vi "delete channel.vi"(10 "Sensor Array":T1, 11 "Indexvals in":u32) -> (2 "Sensor Array out":T1, 3 "Indexvals out":u32)   [LabVIEW 2010]
uses:
  DAQ configuration/Sensor array.ctl
  DAQ configuration/channel identifier.ctl
  global scale array.vi
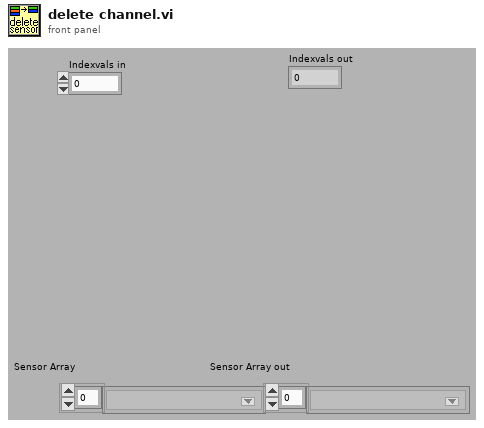
[diagram p1: front panel]
types:
  T1 = typedef "Sensor array.ctl" = T2[]
  T2 = typedef "channel identifier.ctl" = u16
  T3 = typedef "calib array.ctl" = T4[]
  T4 = typedef "conversion.ctl" = cluster{"conversion matrix":sgl[][], "units":string, "name":string, "scale type":T5, "offset (volts)":dbl, "second channel":i8, "correspondence table":T6, "offset (physical units)":dbl, "pH scale":T7, "D.O.":T8}
  T5 = typedef "scale type.ctl" = enum16{"Volts", "Polynomial", "Correspondence Table", "pH", "Dissolved Oxygen", "Quadratic"}
  T6 = typedef "correspondence table.ctl" = cluster{"physical units":dbl, "volts":dbl}[]
  T7 = typedef "pH scale.ctl" = cluster{"Buffers":cluster{"Buffer":dbl, "Calibrated":bool, "V/T":dbl}[], "Temperature":dbl}
  T8 = typedef "DO scale.ctl" = cluster{"Temperature":dbl, "K":dbl, "barometric pressure":dbl}
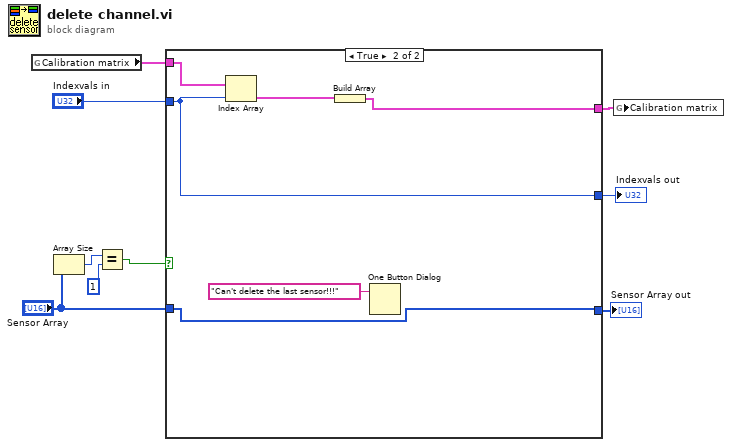
[diagram p0: block diagram]
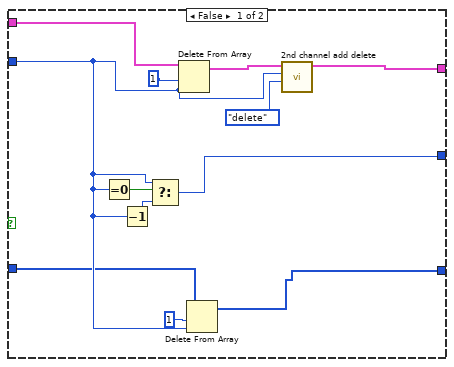
[diagram p2: hidden frame]
diagram:
  n1 = global read "global scale array.vi" "Calibration matrix"() -> (w2:T3)
  n2 = Array Size(array="Sensor Array") -> (size(s)=w6:i32)
  n3 = Equal?(x=w6, y=1) -> (x = y?=w4:bool)
  n4 = case shown="True" w4 {
    tunnel: "Indexvals in" -> [w16 w24]
    tunnel: [w14 w24] -> w8
    tunnel: "Sensor Array" -> [w13 w26]
    tunnel: [w12 w26] -> w3
    tunnel: w2 -> [w11 w25]
    tunnel: [w10 w22] -> w1
    frame False {
      n5 = Equal To 0?(x=w16) -> (x = 0?=w17:bool)
      n6 = Decrement(x=w16) -> (x-1=w15:u32)
      n7 = Select(t=w16, s=w17, f=w15) -> (s? t:f=w14:u32)
      n8 = Delete From Array(array=w11, length=1 ("Length"), index=w16) -> (array with subset deleted=w19:T3)  [unwired: 1 out]
      n9 = Delete From Array(array=w13, length=1 ("Length"), index=w16) -> (array with subset deleted=w12:T1)  [unwired: 1 out]
      n10 = call "2nd channel add delete.vi"("action"=enum16{"delete", "insert"}."delete", "Index"=w16, "Calibration array"=w19) -> ("Calibration array out"=w10:T3)  [unwired: 8 in]
    }
    frame True {
      n11 = Index Array(array=w25, index=w24) -> (element=w23:T4)
      n12 = Build Array(w23) -> (w22:T4[])
      n13 = One Button Dialog(message="Can't delete the last sensor!!!") -> ()  [unwired: 1 in, 1 out]
    }
  }
  "Indexvals out" <- w8
  "Sensor Array out" <- w3
  n14 = global write "global scale array.vi" "Calibration matrix"(w1) -> ()
